vi "Test Configure.vi"(0 "Template RF Test in":refnum<class "niDTS GNSS RF Test.lvclass">, 11 "error in (no error)":errorcluster) -> (4 "Template RF Test out":refnum<class "niDTS GNSS RF Test.lvclass">, 15 "error out":errorcluster)   [LabVIEW 2015, in "niDTS GNSS.lvlib" / "niDTS GNSS RF Test.lvclass"]
uses:
  niDTS GNSS RF Test.lvclass
  Dut/Includes/niDTS GNSS Dut INC Parameters.ctl
  niDTS GNSS RF Test.lvclass/niDTS GNSS RF Test.ctl
  RiviInstDriver/InstDriver/Objects/InstDriver.lvclass/InstDriver.ctl
  RiviInstDriver/InstDriver/Objects/Set VISA Read (Byte Count).vi
  RiviInstDriver/InstDriver/Objects/Read VISA resource.vi
  TestStand/Station/Objects/SystemTechnologyCatalog/niDTS SystemTechnologyCatalog.lvclass
  TestStand/Station/Objects/SystemDut/niDTS SystemDut.lvclass
  Framework/Dut/Objects/BASE_class/niDTS Dut.lvclass
  RiviInstDriver/niRfsgGprf/Objects/niRfsgGprf.lvclass
  TestStand/niDTS TestStand.lvlib
  Framework/niDTS Framework.lvlib
  RiviInstDriver/InstDriver/Objects/InstDriver.lvclass
  niDTS GNSS.lvlib
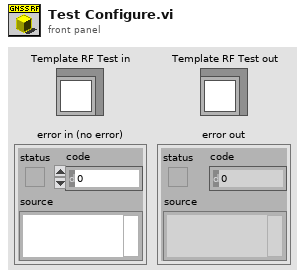
[diagram p1: front panel]
types:
  T1 = typedef "niDTS GNSS.lvlib/niDTS GNSS Dut INC Parameters.ctl" = cluster{"GNSS Standard":enum16{"GPS", "GLONASS", "Galileo", "Beidou"}, "Frequency (Hz)":dbl, "Power (dBm)":dbl, "External Attenuation (dB)":dbl, "Measurement Interval (s)":dbl, "Enable Averaging":bool, "Type Of Averaging":enum16{"MEAN", "MAX", "MIN", "MAXMIN"}, "Number of Averages":i32, "Enable Traces?":bool}
  T2 = typedef "niDTS Framework.lvlib/niDTS Dut INC Handle.ctl" = refnum<data-value>
  T3 = typedef "InstDriver.lvclass/niInstDriver INC Handle.ctl" = refnum<data-value>
  T4 = typedef "niDTS GNSS.lvlib/niDTS GNSS RF Test INC Parameters.ctl" = cluster{"GNSS Standard":enum16{"GPS", "GLONASS", "Galileo", "Beidou"}, "Frequency (Hz)":dbl, "Auto Level":bool, "Power (dBm)":dbl, "External Attenuation (dB)":dbl, "Measurement Interval (s)":dbl, "Pattern":enum16{"0", "1", "01", "00001111", "PN9"}, "Enable Averaging":bool, "Type Of Averaging":enum16{"MEAN", "MAX", "MIN", "MAXMIN"}, "Number of Averages":i32, "Waveform Name":string, "Enable Traces":bool}
  T5 = cluster{"WaveformFileName":string, "WaveformList":string[]}
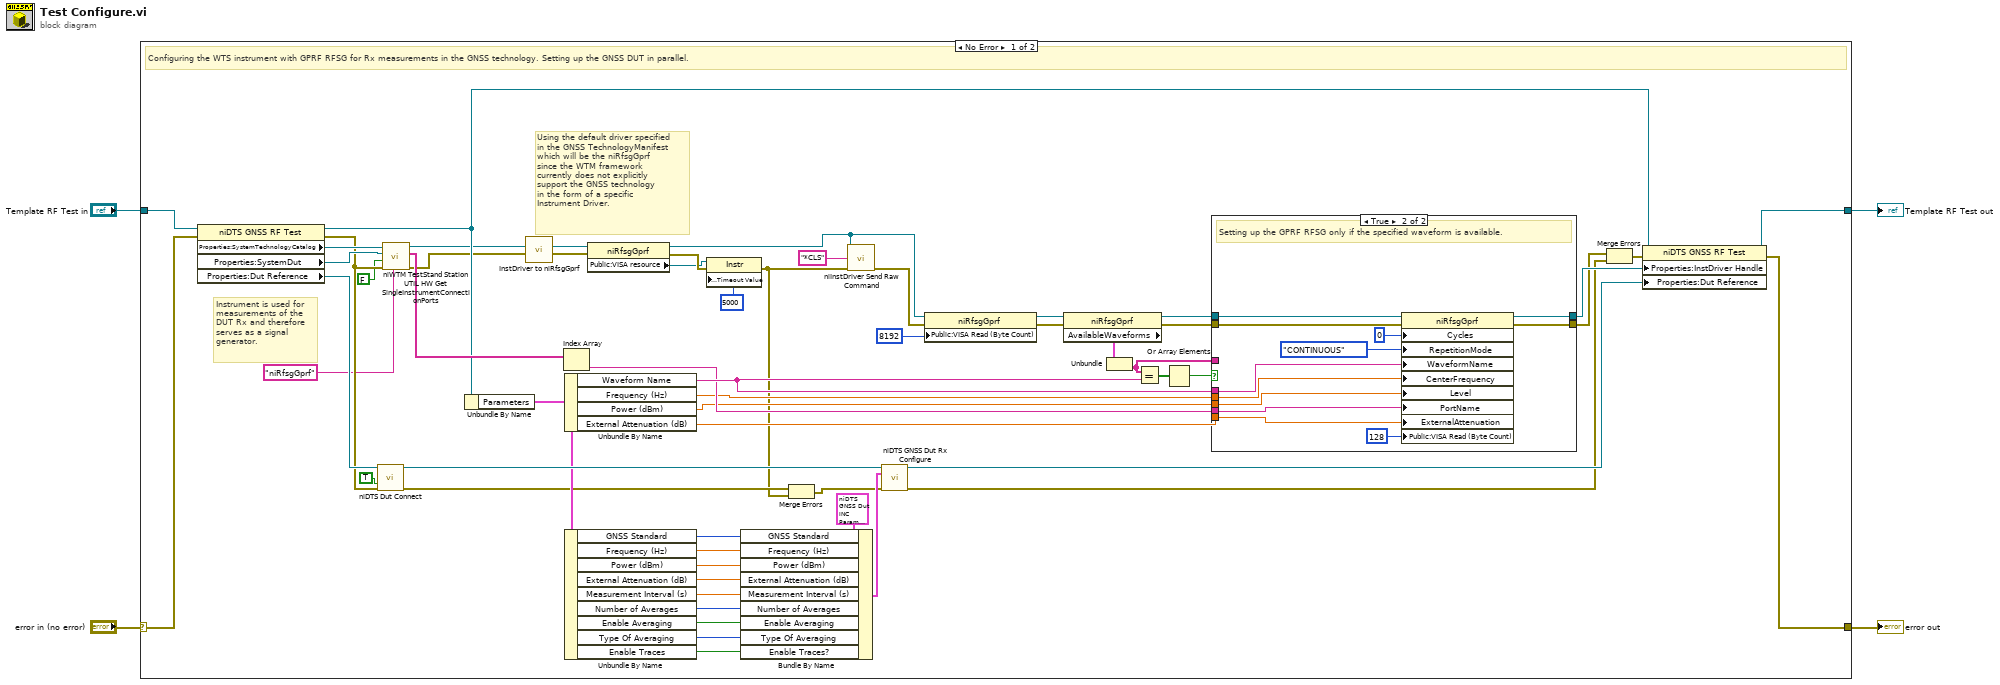
[diagram p0: block diagram]
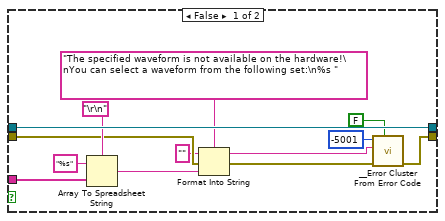
[diagram p2: hidden frame]
diagram:
  n1 = case shown="No Error" "error in (no error)" {
    selector: "error in (no error)" -> [w58 w89]
    tunnel: [w56 w89] -> w2
    tunnel: [w57 w88] -> w3
    tunnel: "Template RF Test in" -> [w62 w88]
    frame No Error {
      # "Instrument is used for \nmeasurements of the \nDUT Rx and therefore \nserves as a signal \ngenerator."
      # "Using the default driver specified\nin the GNSS TechnologyManifest \nwhich will be the niRfsgGprf\nsince the WTM framework \ncurrently does not explicitly \nsupport the GNSS technology\nin the form of a specific \nInstrument Driver."
      # "Configuring the WTS instrument with GPRF RFSG for Rx measurements in the GNSS technology. Setting up the GNSS DUT in parallel."
      n2 = property class="niDTS GNSS RF Test"(reference=w62, error in=w58) -> (reference out=w54:refnum<class "niDTS GNSS RF Test.lvclass">, error out=w8:errorcluster, "Properties:SystemTechnologyCatalog"=w10:refnum<class "niDTS SystemTechnologyCatalog.lvclass">, "Properties:SystemDut"=w9:refnum<class "niDTS SystemDut.lvclass">, "Properties:Dut Reference"=w55:T2)
      n3 = call "niDTS Dut Connect.vi"("Dut Handle"=w55, "Auto Interface"=TRUE, "error in (no error)"=w8) -> ("Dut Handle out"=w60:T2, "error out"=w21:errorcluster)  [unwired: 11 in]
      n4 = call "niWTM TestStand Station UTIL HW Get SingleInstrumentConnectionPorts.vi"("InstDriver Name"="niRfsgGprf", "error in (no error)"=w8, "TX Instrument"=FALSE, "SystemDut"=w9, "SystemTechnologyCatalog"=w10) -> ("error out"=w6:errorcluster, "Ports"=w59:string[], "InstDriver Handle"=w13:T3)  [unwired: 4 in]
      n5 = Unbundle By Name(w54) -> ("Parameters"=w34:T4)
      n6 = call "InstDriver to niRfsgGprf.vi"("error in (no error)"=w6, "InstDriver Handle in"=w13) -> ("error out"=w12:errorcluster, "InstDriver Handle out"=w11:refnum<data-value>)  [unwired: 8 in]
      n7 = Index Array(array=w59) -> (element=w32:string)  [unwired: 1 in]
      n8 = Unbundle By Name(w34) -> ("Waveform Name"=w33:string, "Frequency (Hz)"=w31:dbl, "Power (dBm)"=w30:dbl, "External Attenuation (dB)"=w29:dbl)
      n9 = Unbundle By Name(w34) -> ("GNSS Standard"=w50:enum16{"GPS", "GLONASS", "Galileo", "Beidou"}, "Frequency (Hz)"=w49:dbl, "Power (dBm)"=w48:dbl, "External Attenuation (dB)"=w47:dbl, "Measurement Interval (s)"=w46:dbl, "Number of Averages"=w45:i32, "Enable Averaging"=w42:bool, "Type Of Averaging"=w41:enum16{"MEAN", "MAX", "MIN", "MAXMIN"}, "Enable Traces"=w24:bool)
      n10 = property class="niRfsgGprf"(reference=w11, error in=w12) -> (reference out=w16:refnum<data-value>, error out=w23:errorcluster, "Public:VISA resource"=w22:refnum<visa-resource-name>)
      n11 = property class="Instr"(reference=w22, error in=w23, "General Settings:Timeout Value"=u32 5000) -> (error out=w19:errorcluster)  [unwired: 1 out]
      n12 = Bundle By Name(cluster=T1 {"GNSS Standard"=enum."GPS", "Frequency (Hz)"=0.0, "Power (dBm)"=0.0, "External Attenuation (dB)"=0.0, "Measurement Interval (s)"=1000.0, "Enable Averaging"=FALSE, "Type Of Averaging"=enum."MEAN", "Number of Averages"=1, "Enable Traces?"=FALSE} ("niDTS GNSS DUT Parameters"), "GNSS Standard"=w50, "Frequency (Hz)"=w49, "Power (dBm)"=w48, "External Attenuation (dB)"=w47, "Measurement Interval (s)"=w46, "Number of Averages"=w45, "Enable Averaging"=w42, "Type Of Averaging"=w41, "Enable Traces?"=w24) -> (w44:T1)
      n13 = Merge Errors(w21, w19) -> (w20:errorcluster)
      n14 = call "niInstDriver Send Raw Command.vi"("InstDriver Handle in"=w16, "Command"="*CLS", "error in (no error)"=w19) -> ("error out"=w15:errorcluster)  [unwired: 11 in, 1 out]
      n15 = call "niDTS GNSS Dut Rx Configure.vi"("Dut Handle in"=w60, "niDTS GNSS DUT Parameters"=w44, "error in (no error)"=w20) -> ("Dut Handle out"=w43:T2, "error out"=w26:errorcluster)  [unwired: 11 in]
      n16 = property class="niRfsgGprf"(reference=w16, error in=w15, "Public:VISA Read (Byte Count)"=u32 8192 ("VISA Read (Byte Count)")) -> (reference out=w18:refnum<data-value>, error out=w17:errorcluster)
      n17 = property class="niRfsgGprf"(reference=w18, error in=w17) -> (reference out=w39:refnum<data-value>, error out=w40:errorcluster, "AvailableWaveforms"=w38:T5)
      n18 = Unbundle(w38) -> ("WaveformList"=w35:string[])  [unwired: 1 out]
      n19 = Equal?(x=w35, y=w33) -> (x = y?=w37:bool[])
      n20 = Or Array Elements(Boolean array=w37) -> (logical OR=w36:bool)
      n21 = case shown="True" w36 {
        tunnel: w40 -> [w66 w85]
        tunnel: w39 -> [w75 w84]
        tunnel: w33 -> [_ w83]
        tunnel: w31 -> [_ w82]
        tunnel: w30 -> [_ w81]
        tunnel: w32 -> [_ w80]
        tunnel: w29 -> [_ w79]
        tunnel: [w75 w78] -> w28
        tunnel: [w74 w77] -> w27
        tunnel: w35 -> [w71 _]
        frame False {
          n22 = Array To Spreadsheet String(delimiter (Tab)="\r\n", array=w71, 3:"%s" ("format string")) -> (spreadsheet string=w67:string)
          n23 = Format Into String(format string="The specified waveform is not available on the hardware!\nYou can select a waveform from the following set:\n%s ", initial string="", error in=w66, w67) -> (resulting string=w64:string, error out=w65:errorcluster)
          n24 = call "__Error Cluster From Error Code.vi"("show call chain? (False)"=FALSE, "error in (no error)"=w65, "error message (\"\")"=w64, "error code (0)"=-5001) -> ("error out"=w74:errorcluster)  [unwired: 5 in]
        }
        frame True {
          # "Setting up the GPRF RFSG only if the specified waveform is available."
          n25 = property class="niRfsgGprf"(reference=w84, error in=w85, "Cycles"=0 ("SOURce:RFSG:GPRF:ARB:Cycles"), "RepetitionMode"=enum16{"CONTINUOUS", "FINITE"}."CONTINUOUS" ("SOURce:RFSG:GPRF:ARB:RepetitionMode"), "WaveformName"=w83, "CenterFrequency"=w82, "Level"=w81, "PortName"=w80, "ExternalAttenuation"=w79, "Public:VISA Read (Byte Count)"=u32 128 ("VISA Read (Byte Count)")) -> (reference out=w78:refnum<data-value>, error out=w77:errorcluster)
        }
      }
      n26 = Merge Errors(w27, w26) -> (w25:errorcluster)
      n27 = property class="niDTS GNSS RF Test"(reference=w54, error in=w25, "Properties:InstDriver Handle"=w28, "Properties:Dut Reference"=w43) -> (reference out=w57:refnum<class "niDTS GNSS RF Test.lvclass">, error out=w56:errorcluster)
    }
    frame Error {
    }
  }
  "error out" <- w2
  "Template RF Test out" <- w3
